vi "批次管理.vi"() -> ()   [LabVIEW 2020]
uses:
  <vilib>/addons/database/NI_Database_API.lvlib
  <vilib>/addons/database/Connection.llb/Conn Execute.vi
  <vilib>/addons/database/Connection.llb/DB Tools Open Connec (String).vi
  <vilib>/addons/database/Recordset.llb/Rec Destroy - Connection.vi
  <vilib>/addons/database/Recordset.llb/Rec Fetch Recordset Data (R).vi
  Global_Variable/Global.vi
panel:
  out "产品型号":string
  out "批次信息":string[][](table)
  # "批次管理"
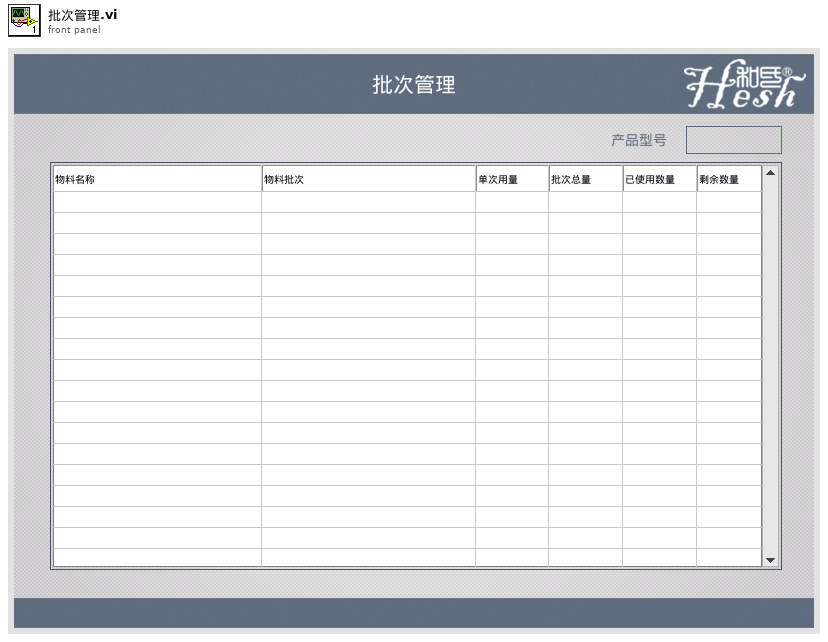
[diagram p1: front panel]
types:
  T1 = typedef "NI_Database_API.lvlib/Conn ObjectReference.ctl" = refnum<k1>
  T2 = typedef "NI_Database_API.lvlib/Rec ObjectReference.ctl" = refnum<k1>
  T3 = typedef "LVPoint32TypeDef.ctl" = cluster{"Horizontal":i32, "Vertical":i32}
  T4 = typedef "LVRowAndColumnTypeDef.ctl" = cluster{"Row":i32, "Column":i32}
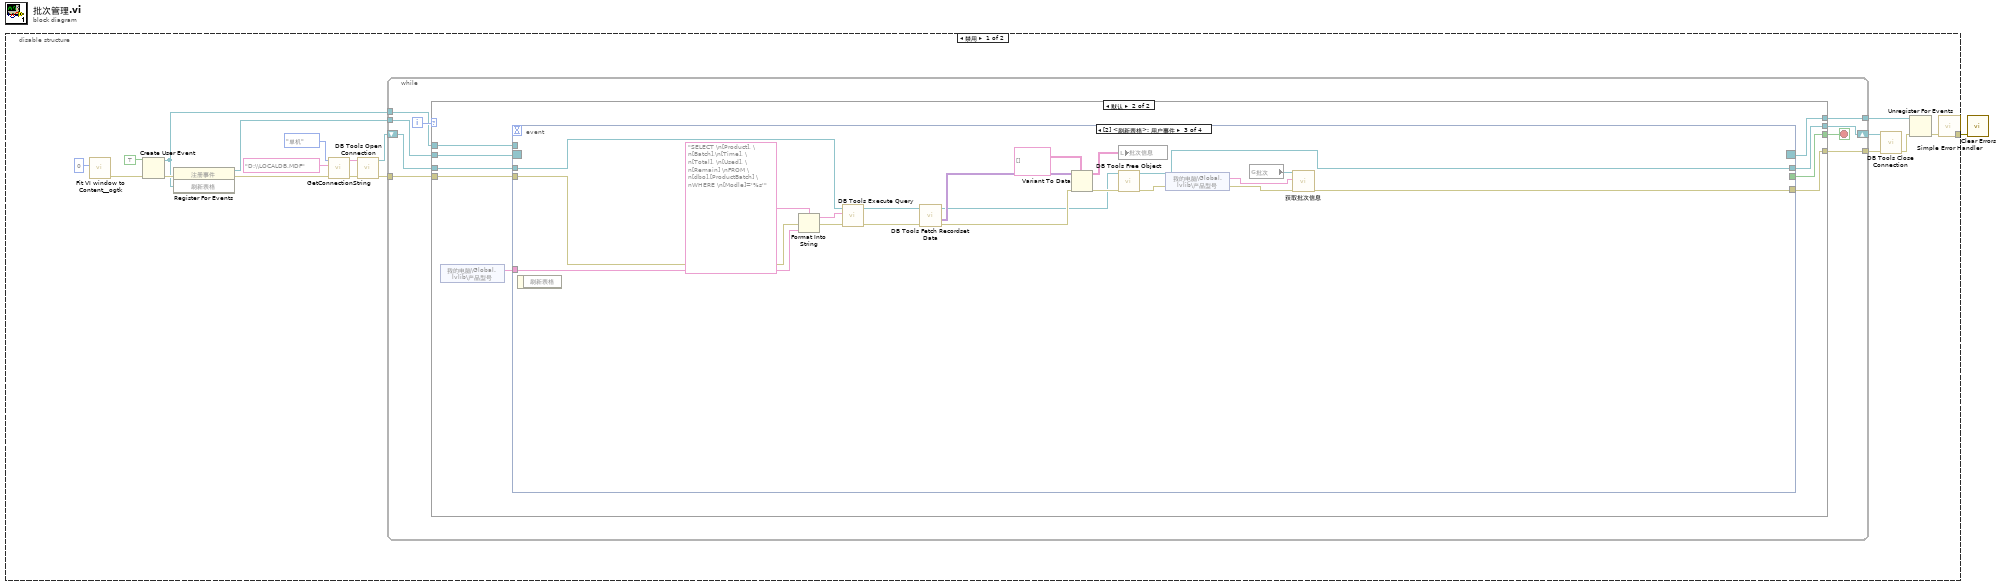
[diagram p0: block diagram]
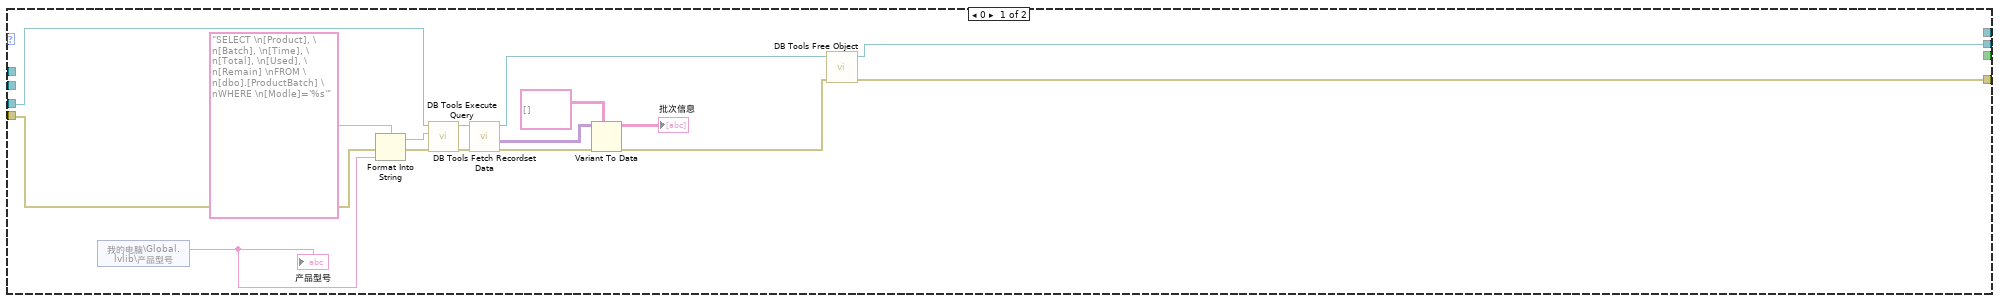
[diagram p2: hidden frame]
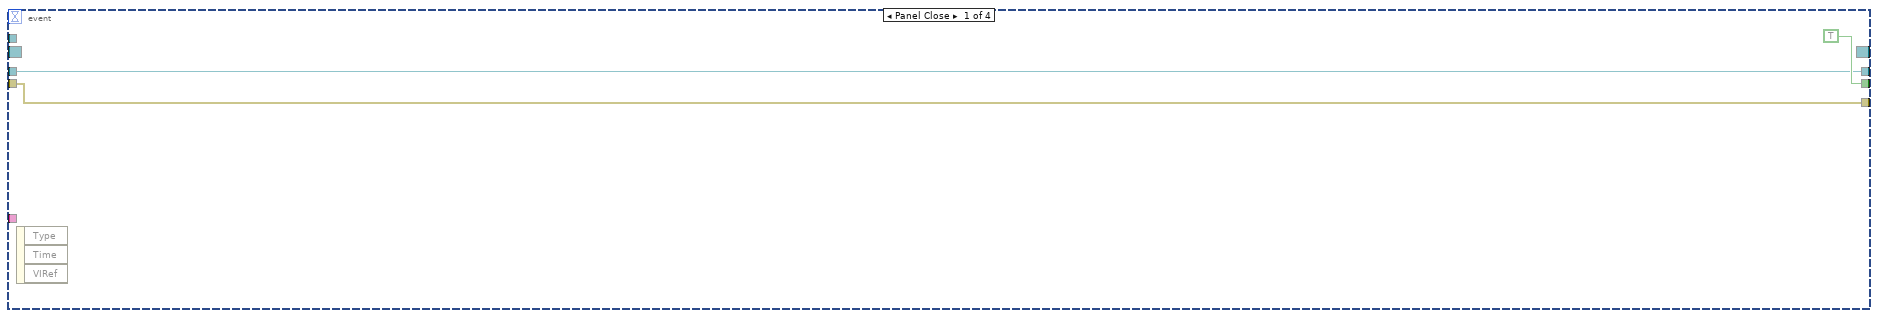
[diagram p3: hidden frame]
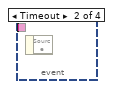
[diagram p4: hidden frame]
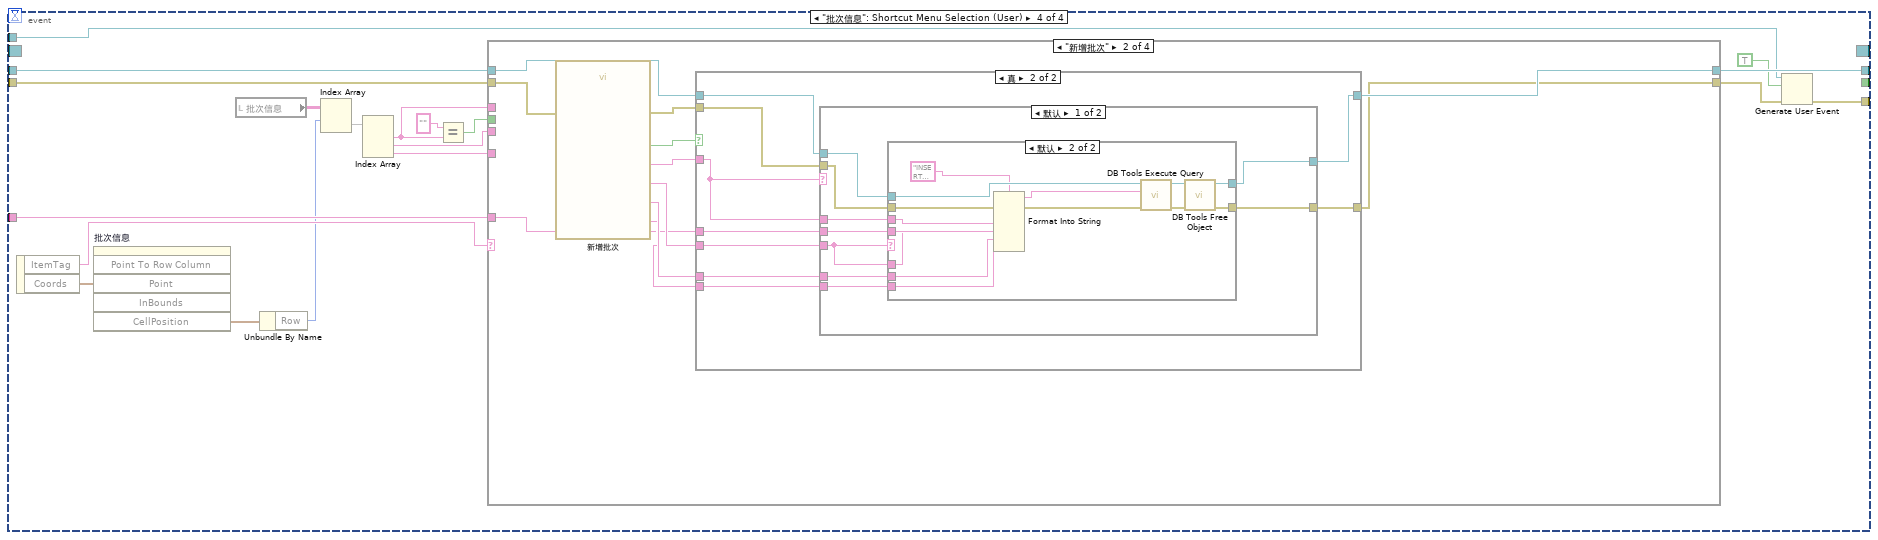
[diagram p5: hidden frame]
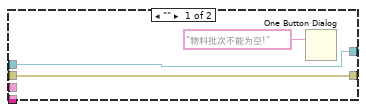
[diagram p8: hidden frame]
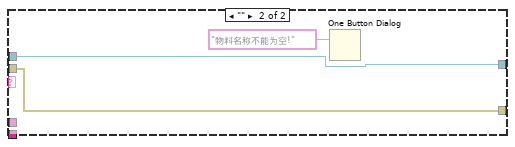
[diagram p9: hidden frame]
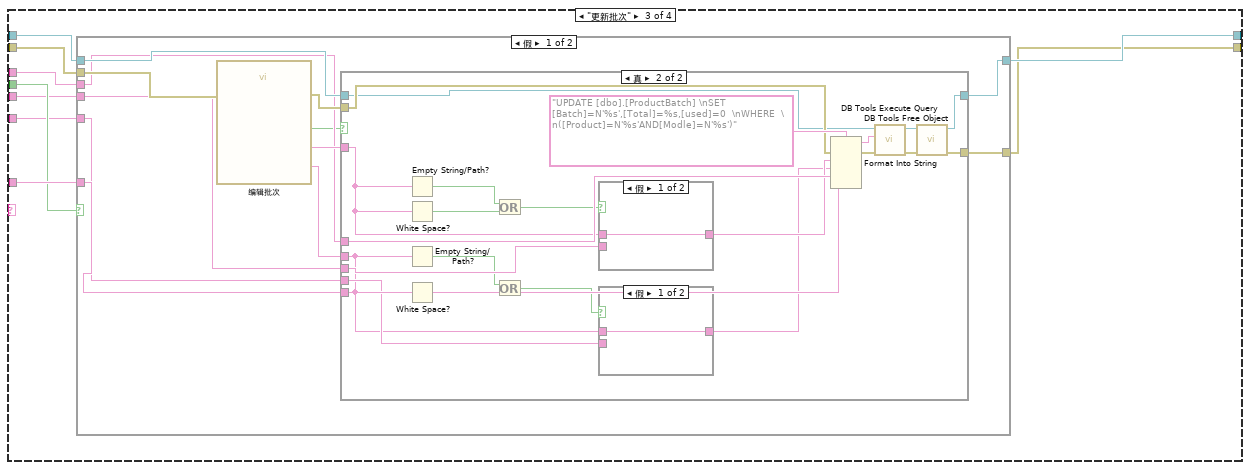
[diagram p10: hidden frame]
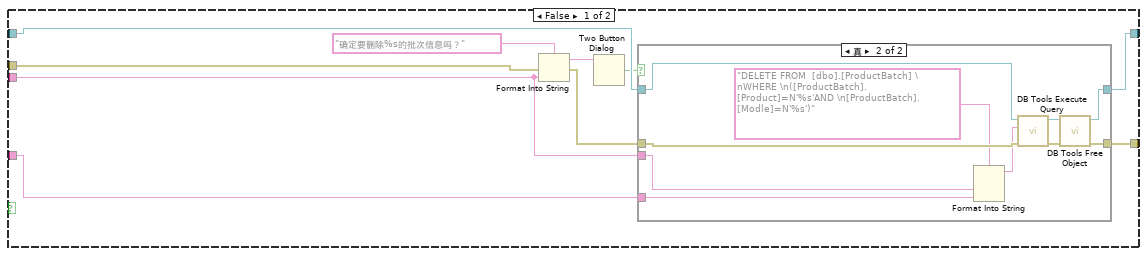
[diagram p16: hidden frame]
diagram:
  n1 = disable-structure shown="禁用" {
    disable-tunnel: [w13 _] -> w1
    frame Disabled {
      n2 = call <userlib>:"Fit VI window to Content__ogtk.vi"("border spacing (2 px)"=0) -> ("error out"=w3:errorcluster)  [unwired: 5 in, 1 out]
      n3 = Create User Event(user event datatype=TRUE ("刷新表格"), error in=w3) -> (user event=w4:refnum<user-event>, error out=w6:errorcluster)
      n4 = register-events(error in=w6, w4) -> (reference out=w12:refnum<event-registration>, error out=w8:errorcluster)  [unwired: 1 in]
      n5 = call "GetConnectionString.vi"("error in (no error)"=w8, "Database Name"="D:\\LOCALDB.MDF", "连接模式"=enum16{"单机", "联网"}."单机") -> ("error out"=w7:errorcluster, "连接字符串"=w20:string)  [unwired: 3 in]
      n6 = call-poly <vilib>:"DB Tools Open Connection.vi"("error in (no error)"=w7, "connection information"=w20) -> ("error out"=w16:errorcluster, "connection reference"=w17:T1)  [unwired: 6 in]
      n7 = while {
        tunnel: w16 -> [w27]
        tunnel: [w25] -> w14
        shift-right: [w26] -> w15
        shift-left: w17 -> [w28]
        tunnel: w12 -> [w24]
        tunnel: [w23] -> w11
        tunnel: w4 -> [w21]
        i -> [w22]
        stop <- w29 stop-if-true
        n8 = case shown="默认" w22 {
          tunnel: [_ w54] -> w29
          tunnel: w28 -> [w31 w53]
          tunnel: w27 -> [w32 w52]
          tunnel: [w34 w51] -> w26
          tunnel: [w33 w50] -> w25
          tunnel: w24 -> [_ w49]
          tunnel: [_ w48] -> w23
          tunnel: w21 -> [_ w47]
          frame 0 {
            n9 = shared-variable "我的电脑\\Global.lvlib\\产品型号"() -> (w30:string)  [unwired: 1 in, 1 out]
            "产品型号" <- w30
            n10 = Format Into String(format string="SELECT \n[Product], \n[Batch], \n[Time], \n[Total], \n[Used], \n[Remain] \nFROM \n[dbo].[ProductBatch] \nWHERE \n[Modle]='%s'" ("格式字符串"), error in=w32, w30) -> (resulting string=w36:string, error out=w37:errorcluster)  [unwired: 1 in]
            n11 = call-poly <vilib>:"DB Tools Execute Query.vi"("error in (no error)"=w37, "SQL query"=w36, "connection reference"=w31) -> ("error out"=w45:errorcluster, "recordset reference"=w44:T2)  [unwired: 5 in]
            n12 = call-poly <vilib>:"DB Tools Fetch Recordset Data.vi"("error in (no error)"=w45, "recordset reference"=w44) -> ("error out"=w43:errorcluster, "recordset data"=w42:variant[][], "recordset reference out"=w39:T2)  [unwired: 3 in]
            n13 = Variant To Data(error in=w43, type=string[][] [], Variant=w42) -> (data=→"批次信息":string[][], error out=w40:errorcluster)
            n14 = call-poly <vilib>:"DB Tools Free Object.vi"("error in (no error)"=w40, "recordset reference"=w39) -> ("error out"=w33:errorcluster, "connection reference"=w34:T1)  [unwired: 8 in]
          }
          frame Default {
            n15 = shared-variable "我的电脑\\Global.lvlib\\产品型号"() -> (w46:string)  [unwired: 1 in, 1 out]
            n16 = event shown="[2] <刷新表格>: 用户事件" {
              selector: w49 -> [_ _ _ _]
              dyn-events: [_ _ _ _] -> w48
              timeout: _ -> [_ _ _ _]
              tunnel: [TRUE _ _ _] -> w54
              tunnel: w53 -> [w56 _ w67 w95]
              tunnel: w52 -> [w55 _ w65 w94]
              tunnel: [w56 _ w64 w93] -> w51
              tunnel: [w55 _ w59 w84] -> w50
              tunnel: w46 -> [_ _ w66 w92]
              tunnel: w47 -> [_ _ _ w87]
              event Panel Close {
                n17 = event-data() -> ()  [unwired: 1 in, 3 out]
              }
              event Timeout {
                n18 = event-data() -> ()  [unwired: 1 in, 1 out]
              }
              event User Event {
                n19 = event-data() -> ()  [unwired: 1 in, 1 out]
                n20 = Format Into String(format string="SELECT \n[Product], \n[Batch],\n[Time], \n[Total], \n[Used], \n[Remain] \nFROM \n[dbo].[ProductBatch] \nWHERE \n[Modle]='%s'" ("格式字符串"), error in=w65, w66) -> (resulting string=w68:string, error out=w69:errorcluster)  [unwired: 1 in]
                n21 = call-poly <vilib>:"DB Tools Execute Query.vi"("error in (no error)"=w69, "SQL query"=w68, "connection reference"=w67) -> ("error out"=w77:errorcluster, "recordset reference"=w76:T2)  [unwired: 5 in]
                n22 = call-poly <vilib>:"DB Tools Fetch Recordset Data.vi"("error in (no error)"=w77, "recordset reference"=w76) -> ("error out"=w75:errorcluster, "recordset data"=w74:variant[][], "recordset reference out"=w71:T2)  [unwired: 3 in]
                n23 = Variant To Data(error in=w75, type=string[][] [], Variant=w74) -> (data=w63:string[][], error out=w72:errorcluster)
                n24 = local write "批次信息"(w63) -> ()
                n25 = call-poly <vilib>:"DB Tools Free Object.vi"("error in (no error)"=w72, "recordset reference"=w71) -> ("error out"=w61:errorcluster, "connection reference"=w64:T1)  [unwired: 8 in]
                n26 = shared-variable "我的电脑\\Global.lvlib\\产品型号"(error in=w61) -> (w62:string, error out=w60:errorcluster)
                n27 = global read "Global.vi" "批次"() -> (w58:refnum<vi>)
                n28 = call "获取批次信息.vi"("error in (no error)"=w60, "产品型号"=w62, "Tbl引用句柄"=w58) -> ("error out"=w59:errorcluster)  [unwired: 7 in, 1 out]
              }
              event "批次信息": Shortcut Menu Selection (User) {
                n29 = event-data() -> ("ItemTag"=w96:string, "Coords"=w83:T3)  [unwired: 1 in]
                n30 = invoke on="批次信息" class="Tbl (严格)" method="Point To Row Column"("Point"=w83) -> ("CellPosition"=w82:T4)  [unwired: 5 in, 5 out]
                n31 = local read "批次信息"() -> (w89:string[][])
                n32 = Unbundle By Name(w82) -> ("Row"=w90:i32)
                n33 = Index Array(array=w89, index (row)=w90) -> (element=w81:string[])  [unwired: 1 in]
                n34 = Index Array(array=w81) -> (element #1=w80:string, element #2=w79:string, element #3=w78:string)  [unwired: 3 in]
                n35 = Equal?(x="" ("元素"), y=w80) -> (x = y?=w88:bool)
                n36 = case shown="\"新增批次\"" w96 {
                  tunnel: w95 -> [w97 w109 w157 w208]
                  tunnel: w94 -> [w98 w106 w156 w207]
                  tunnel: [w98 w107 w152 w203] -> w85
                  tunnel: [w97 w108 w153 w204] -> w93
                  tunnel: w92 -> [_ w99 w158 w205]
                  tunnel: w80 -> [_ _ w154 w206]
                  tunnel: w88 -> [_ _ w155 w202]
                  tunnel: w79 -> [_ _ w151 _]
                  tunnel: w78 -> [_ _ w150 _]
                  frame Default {
                  }
                  frame "新增批次" {
                    n37 = call "新增批次"("error in (no error)"=w106) -> ("单次使用数量"=w100:string, "批次数量"=w102:string, "物料批次"=w103:string, "物料名称"=w104:string, "确定"=w105:bool, "error out"=w101:errorcluster)  [unwired: 13 in]
                    n38 = case shown="真" w105 {
                      tunnel: [w110 w120] -> w107
                      tunnel: [w111 w119] -> w108
                      tunnel: w104 -> [_ w113]
                      tunnel: w103 -> [_ w114]
                      tunnel: w102 -> [_ w118]
                      tunnel: w109 -> [w111 w117]
                      tunnel: w101 -> [w110 w116]
                      tunnel: w99 -> [_ w115]
                      tunnel: w100 -> [_ w112]
                      frame False {
                      }
                      frame True {
                        n39 = case shown="默认" w113 {
                          tunnel: [w129 w148] -> w120
                          tunnel: [w128 w149] -> w119
                          tunnel: w118 -> [w127 _]
                          tunnel: w117 -> [w126 w149]
                          tunnel: w116 -> [w125 w148]
                          tunnel: w115 -> [w124 _]
                          tunnel: w113 -> [w123 _]
                          tunnel: w114 -> [w122 _]
                          tunnel: w112 -> [w121 _]
                          frame Default {
                            n40 = case shown="默认" w122 {
                              tunnel: [w130 w142] -> w129
                              tunnel: [w131 w141] -> w128
                              tunnel: w127 -> [_ w140]
                              tunnel: w126 -> [w131 w139]
                              tunnel: w125 -> [w130 w138]
                              tunnel: w124 -> [_ w137]
                              tunnel: w123 -> [_ w136]
                              tunnel: w122 -> [_ w135]
                              tunnel: w121 -> [_ w133]
                              frame "" {
                                n41 = One Button Dialog(message="物料批次不能为空!" ("消息")) -> ()  [unwired: 1 in, 1 out]
                              }
                              frame Default {
                                n42 = Format Into String(format string="INSERT INTO \n[dbo].[ProductBatch] \n([Modle], [Product],[Batch],[Total],[Time]) \nVALUES (N'%s',N'%s', N'%s',N'%s',N'%s')" ("格式字符串"), error in=w138, w137, w136, w135, w140, w133) -> (resulting string=w146:string, error out=w143:errorcluster)  [unwired: 1 in]
                                n43 = call-poly <vilib>:"DB Tools Execute Query.vi"("error in (no error)"=w143, "SQL query"=w146, "connection reference"=w139) -> ("error out"=w145:errorcluster, "recordset reference"=w144:T2)  [unwired: 5 in]
                                n44 = call-poly <vilib>:"DB Tools Free Object.vi"("error in (no error)"=w145, "recordset reference"=w144) -> ("error out"=w142:errorcluster, "connection reference"=w141:T1)  [unwired: 8 in]
                              }
                            }
                          }
                          frame "" {
                            n45 = One Button Dialog(message="物料名称不能为空!" ("消息")) -> ()  [unwired: 1 in, 1 out]
                          }
                        }
                      }
                    }
                  }
                  frame "更新批次" {
                    n46 = case shown="假" w155 {
                      tunnel: w158 -> [w165 _]
                      tunnel: w157 -> [w169 w200]
                      tunnel: w156 -> [w168 w201]
                      tunnel: w154 -> [w166 _]
                      tunnel: [w164 w200] -> w153
                      tunnel: [w163 w201] -> w152
                      tunnel: w151 -> [w161 _]
                      tunnel: w150 -> [w160 _]
                      frame False {
                        n47 = call "编辑批次"("error in (no error)"=w168) -> ("批次数量"=w159:string, "物料批次"=w167:string, "确定"=w162:bool, "error out"=w170:errorcluster)  [unwired: 15 in]
                        n48 = case shown="真" w162 {
                          tunnel: w169 -> [w172 w187]
                          tunnel: w170 -> [w171 w190]
                          tunnel: w159 -> [_ w174]
                          tunnel: [w172 w189] -> w164
                          tunnel: [w171 w188] -> w163
                          tunnel: w167 -> [_ w180]
                          tunnel: w166 -> [_ w186]
                          tunnel: w165 -> [_ w185]
                          tunnel: w161 -> [_ w183]
                          tunnel: w160 -> [_ w182]
                          frame False {
                          }
                          frame True {
                            n49 = Empty String/Path?(string/path=w180) -> (empty?=w179:bool)
                            n50 = White Space?(1:w180) -> (0:w178:bool)
                            n51 = Empty String/Path?(string/path=w174) -> (empty?=w176:bool)
                            n52 = White Space?(1:w174) -> (0:w175:bool)
                            n53 = Or(x=w179, y=w178) -> (x .or. y?=w177:bool)
                            n54 = Or(x=w176, y=w175) -> (x .or. y?=w173:bool)
                            n55 = case shown="假" w177 {
                              tunnel: w180 -> [w198 _]
                              tunnel: [w198 w199] -> w184
                              tunnel: w183 -> [_ w199]
                              frame False {
                              }
                              frame True {
                              }
                            }
                            n56 = case shown="假" w173 {
                              tunnel: w174 -> [w196 _]
                              tunnel: [w196 w197] -> w181
                              tunnel: w182 -> [_ w197]
                              frame False {
                              }
                              frame True {
                              }
                            }
                            n57 = Format Into String(format string="UPDATE [dbo].[ProductBatch] \nSET [Batch]=N'%s',[Total]=%s,[used]=0  \nWHERE  \n([Product]=N'%s'AND[Modle]=N'%s')" ("格式字符串"), error in=w190, w184, w181, w186, w185) -> (resulting string=w194:string, error out=w191:errorcluster)  [unwired: 1 in]
                            n58 = call-poly <vilib>:"DB Tools Execute Query.vi"("error in (no error)"=w191, "SQL query"=w194, "connection reference"=w187) -> ("error out"=w193:errorcluster, "recordset reference"=w192:T2)  [unwired: 5 in]
                            n59 = call-poly <vilib>:"DB Tools Free Object.vi"("error in (no error)"=w193, "recordset reference"=w192) -> ("error out"=w188:errorcluster, "connection reference"=w189:T1)  [unwired: 8 in]
                          }
                        }
                      }
                      frame True {
                      }
                    }
                  }
                  frame "删除批次" {
                    n60 = case shown="真" w202 {
                      tunnel: w206 -> [w210 _]
                      tunnel: w207 -> [w217 w231]
                      tunnel: w208 -> [w215 w232]
                      tunnel: [w213 w232] -> w204
                      tunnel: [w212 w231] -> w203
                      tunnel: w205 -> [w209 _]
                      frame False {
                        n61 = Format Into String(format string="确定要删除%s的批次信息吗？" ("格式字符串"), error in=w217, w210) -> (resulting string=w216:string, error out=w214:errorcluster)  [unwired: 1 in]
                        n62 = Two Button Dialog(message=w216) -> (T button?=w211:bool)  [unwired: 2 in]
                        n63 = case shown="真" w211 {
                          tunnel: w215 -> [w220 w230]
                          tunnel: w214 -> [w219 w229]
                          tunnel: [w220 w226] -> w213
                          tunnel: [w219 w225] -> w212
                          tunnel: w210 -> [_ w223]
                          tunnel: w209 -> [_ w221]
                          frame False {
                          }
                          frame True {
                            n64 = Format Into String(format string="DELETE FROM  [dbo].[ProductBatch] \nWHERE \n([ProductBatch].[Product]=N'%s'AND \n[ProductBatch].[Modle]=N'%s')" ("格式字符串"), w223, w221) -> (resulting string=w222:string)  [unwired: 2 in, 1 out]
                            n65 = call-poly <vilib>:"DB Tools Execute Query.vi"("error in (no error)"=w229, "SQL query"=w222, "connection reference"=w230) -> ("error out"=w228:errorcluster, "recordset reference"=w227:T2)  [unwired: 5 in]
                            n66 = call-poly <vilib>:"DB Tools Free Object.vi"("error in (no error)"=w228, "recordset reference"=w227) -> ("error out"=w225:errorcluster, "connection reference"=w226:T1)  [unwired: 8 in]
                          }
                        }
                      }
                      frame True {
                      }
                    }
                  }
                }
                n67 = Generate User Event(user event=w87, event data cluster=TRUE ("事件数据"), error in=w85) -> (error out=w84:errorcluster)  [unwired: 1 in, 1 out]
              }
            }
          }
        }
      }
      n68 = call <vilib>:"DB Tools Close Connection.vi"("error in (no error)"=w14, "connection reference"=w15) -> ("error out"=w10:errorcluster)  [unwired: 5 in]
      n69 = Unregister For Events(event registration refnum=w11, error in=w10) -> (error out=w9:errorcluster)
      n70 = call <vilib>:"Simple Error Handler.vi"("error in (no error)"=w9) -> ("error out"=w13:errorcluster)  [unwired: 4 in, 4 out]
    }
    frame Enabled {
    }
  }
  n71 = call <vilib>:"Clear Errors.vi"("error in (no error)"=w1) -> ()  [unwired: 5 in, 2 out]
